vi "Check If Parent Missile.vi"(9 "GB Components in":refnum<class "Game Board Component.lvclass">[](array[class]), 11 "Game Board Component in":refnum<class "Game Board Component.lvclass">) -> (2 "Not parent missile?":bool)   [LabVIEW 2021, in "Game Board Component.lvclass"]
doc: "MIT Licence\nCopyright (c) 2024 David Grollier"
uses:
  Game Board Component.lvclass
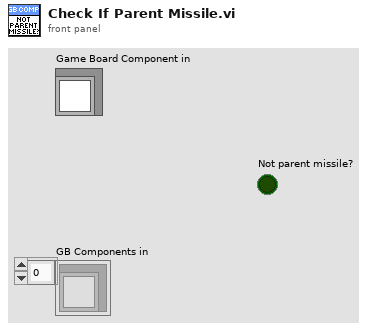
[diagram p1: front panel]
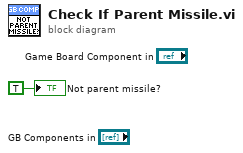
[diagram p0: block diagram]
diagram:
  "Not parent missile?" <- TRUE ("Not parent missile?")
